vi "SubVI_Open_Save_Folder.vi"(8 "error in (no error)":errorcluster, 11 "Save Folder Path":path) -> (0 "error out":errorcluster, 3 "Resulting Folder Path":path)   [LabVIEW 2020]
uses:
  Global 1.vi
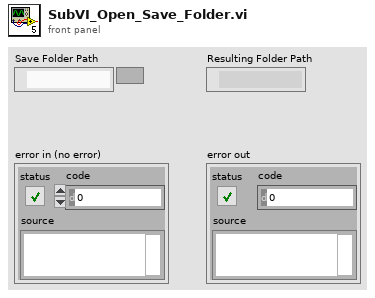
[diagram p1: front panel]
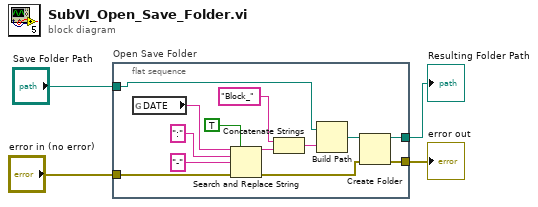
[diagram p0: block diagram]
diagram:
  n1 = flat-sequence "Open Save Folder" {
    tunnel: [w14] -> w1
    tunnel: "error in (no error)" -> [w8]
    tunnel: [w7] -> w3
    tunnel: "Save Folder Path" -> [w5]
    frame #0 {
      n2 = global read "Global 1.vi" "DATE"() -> (w6:string)
      n3 = Search and Replace String(replace all?=TRUE ("replace all? (F)"), input string=w6, search string=":" ("input string"), replace string="-" ("replace string (\"\")"), error in=w8) -> (result string=w10:string, error out=w11:errorcluster)  [unwired: 3 in, 2 out]
      n4 = Concatenate Strings("Block_" ("string"), w10) -> (w15:string)
      n5 = Build Path(base path=w5, name or relative path=w15) -> (appended path=w17:path)
      n6 = Create Folder(path (use dialog)=w17, error in=w11) -> (created path=w14:path, error out=w7:errorcluster)  [unwired: 1 in, 1 out]
    }
  }
  "error out" <- w3
  "Resulting Folder Path" <- w1
